vi "mainVI.vi"() -> ()   [LabVIEW 2017]
uses:
  Controls/DataCluster.ctl
panel:
  in  "init":bool
  in  "SP":dbl
  out "CV":dbl
  out "Waveform Chart":cluster{"P1":dbl, "P2":dbl, "P3":dbl}(graph)
  in  "NIS":u32
  in  "Dt":u32
  in  "Stop Button":bool
  in  "P0":dbl(slide) scale=0.0..10.0 scale format="%#_6p"
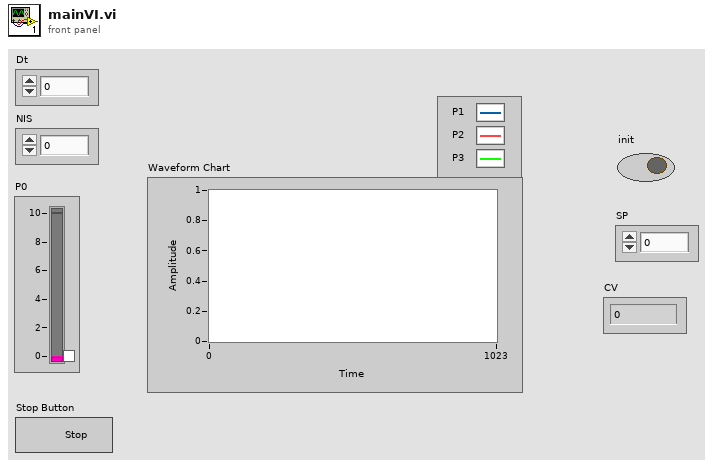
[diagram p1: front panel]
types:
  T1 = enum16{"open", "replace", "create", "open or create", "replace or create", "replace or create with confirmation"}
  T2 = typedef "DataCluster.ctl" = cluster{"P1":dbl, "P2":dbl, "P3":dbl}
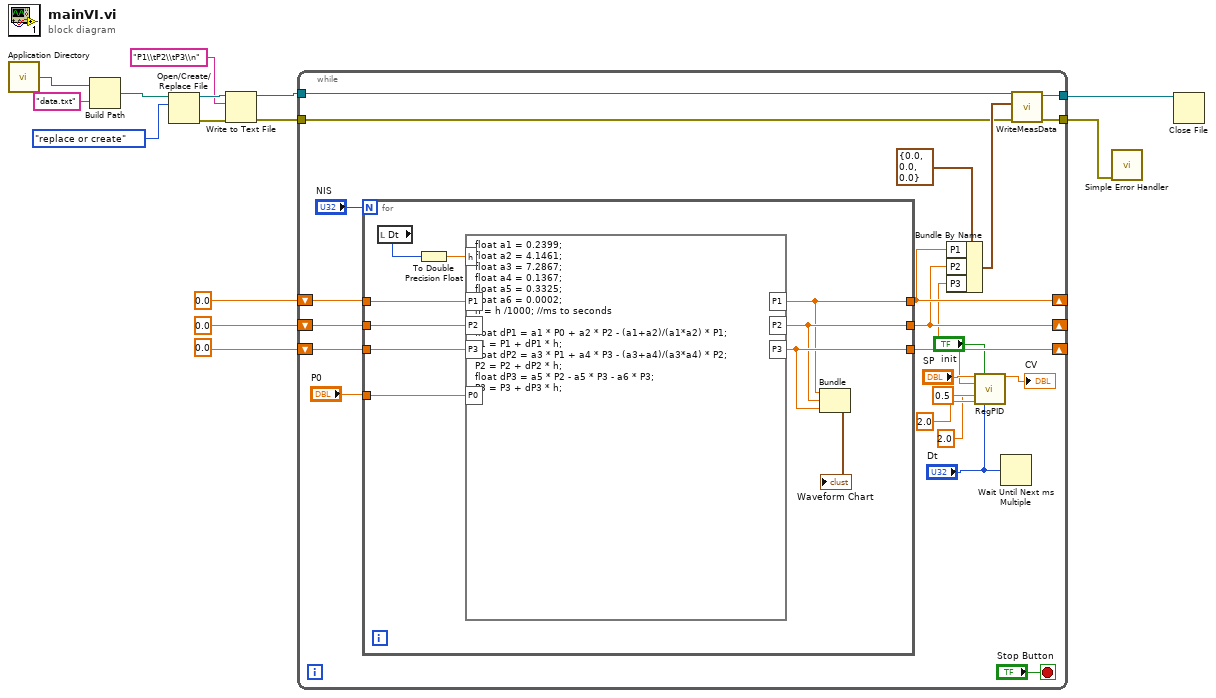
[diagram p0: block diagram]
diagram:
  n1 = call <vilib>:"Application Directory.vi"() -> ("Application Directory"=w9:path)
  n2 = Build Path(base path=w9, name or relative path="data.txt") -> (appended path=w8:path)
  n3 = Open/Create/Replace File(file path (use dialog)=w8, operation (0:open)=T1."replace or create") -> (refnum out=w5:refnum<file>, error out=w2:errorcluster)  [unwired: 4 in, 1 out]
  n4 = Write to Text File(file (use dialog)=w5, text="P1\\tP2\\tP3\\n", error in=w2) -> (refnum out=w4:refnum<file>, error out=w3:errorcluster)  [unwired: 1 in, 1 out]
  n5 = while {
    shift-right: [w31] -> _
    shift-left: 0.0 -> [w35]
    shift-right: [w24] -> _
    shift-left: 0.0 -> [w34]
    shift-right: [w21] -> _
    shift-left: 0.0 -> [w33]
    tunnel: w4 -> [w29]
    tunnel: [w28] -> w10
    tunnel: w3 -> [w26]
    tunnel: [w25] -> w6
    stop <- "Stop Button" stop-if-true
    n6 = for {
      N: "NIS" -> [_]
      tunnel: "P0" -> [w46]
      tunnel: w35 -> [w45]
      tunnel: w34 -> [w44]
      tunnel: w33 -> [w43]
      tunnel: [w40] -> w31
      tunnel: [w41] -> w24
      tunnel: [w42] -> w21
      n7 = local read "Dt"() -> (w38:u32)
      n8 = To Double Precision Float(number=w38) -> (double precision float=w37:dbl)
      n9 = formula code="float a1 = 0.2399;\nfloat a2 = 4.1461;\nfloat a3 = 7.2867;\nfloat a4 = 0.1367;\nfloat a5 = 0.3325;\nfloat a6 = 0.0002;\nh = h /1000; //ms to seconds\n\nfloat dP1 = a1 * P0 + a2 * P2 - (a1+a2)/(a1*a2) * P1;\nP1 = P1 + dP1 * h;\nfloat dP2 = a3 * P1 + a4 * P3 - (a3+a4)/(a3*a4) * P2;\nP2 = P2 + dP2 * h;\nfloat dP3 = a5 * P2 - a5 * P3 - a6 * P3;\nP3 = P3 + dP3 * h;"("P0"=w46, "P1"=w45, "P2"=w44, "P3"=w43, "h"=w37) -> ("P1"=w40:dbl, "P2"=w41:dbl, "P3"=w42:dbl)
      n10 = Bundle("P1"=w40, "P2"=w41, "P3"=w42) -> (→"Waveform Chart":cluster{"P1":dbl, "P2":dbl, "P3":dbl})  [unwired: 1 in]
    }
    n11 = Bundle By Name(cluster=T2 {"P1"=0.0, "P2"=0.0, "P3"=0.0} ("Cluster"), "P1"=w31, "P2"=w24, "P3"=w21) -> (w27:T2)
    n12 = call "RegPID.vi"("SP"="SP", "init"="init", "PV"=w21, "kr"=0.5, "TI"=2.0, "TD"=2.0, "h"="Dt") -> ("CV"=→"CV":dbl)  [unwired: 8 in]
    n13 = Wait Until Next ms Multiple(millisecond multiple="Dt") -> ()  [unwired: 1 out]
    n14 = call "WriteMeasData.vi"("error in (no error)"=w26, "Data Cluster"=w27, "Byte Stream File in"=w29) -> ("error out"=w25:errorcluster, "Byte Stream File out"=w28:refnum<file>)  [unwired: 7 in]
  }
  n15 = call <vilib>:"Simple Error Handler.vi"("error in (no error)"=w6) -> ()  [unwired: 4 in, 5 out]
  n16 = Close File(refnum=w10) -> ()  [unwired: 1 in, 2 out]
